vi "Workspace Tool with Event Messages - Starting point.vi"() -> ()   [LabVIEW 2016]
uses:
  NationalInstruments.VeriStand.SystemStorageUI
  NationalInstruments.VeriStand.SystemStorage
  <vilib>/NI Veristand/Templates/Workspace Tool Support/Workspace Tool Message Bus.ctl
  <vilib>/NI Veristand/Templates/Workspace Tool Support/Workspace Tool Message (String).ctl
  <vilib>/NI Veristand/Templates/Workspace Tool Support/Workspace Tool Response (String).ctl
  <vilib>/NI Veristand/Templates/Workspace Tool Support/Workspace Tool Message (Byte Array).ctl
  <vilib>/NI Veristand/Templates/Workspace Tool Support/Workspace Tool Response (Byte Array).ctl
  <vilib>/NI Veristand/Execution/Workspace/NI VeriStand - Get Multiple Channel Values.vi
  <vilib>/NI VeriStand/Execution/Workspace/NI_VS Workspace ExecutionAPI.lvlib
  <vilib>/NI Veristand/UI Controls/Single Node Browser/NI_VS UI Single Node Browser.lvlib
  <vilib>/NI VeriStand/Templates/Workspace Tool Support/NI VeriStand - Workspace Tool Support.lvlib
  <vilib>/NI Veristand/UI Controls/System Definition Tree/NI_VS UI System Tree.lvlib
panel:
  out "x+1":i32
  out "size(s)":i32
  out "types":i32[](array[ring]) items=["K_STRING", "K_BOOL", "K_I32", "K_U32", "K_DOUBLE", "K_U64", "K_VARIANT", "K_DEPENDENTFILE", "K_DEPENDENTNODE", "K_DATASOURCENODE", "K_U16", "K_DBLARR", "K_U32ARR", "K_I32ARR", "K_STRINGARR", "K_DICTIONARY", "K_DICTIONARYARR", "K_BINARYSTRING", "K_I16", "K_I64", "K_BOOLARR", "K_U64ARR", "K_U16ARR", "K_I64ARR", "K_I16ARR"]
  out "names":string[](array[string])
  in  "NIVS.Message Bus":T1
  out "Byte Array Data":u8[](array[numeric])
  out "String Data":string
  in  "Stop":bool
  in  "NIVS.System Definition Root":refnum<k24>
  in  "Tree Browser":refnum<k24>(container)
  in  "NIVS.Project File Path":path
  in  "Single Node Browser":refnum<k24>(container)
  in  "NIVS.Workspace Event":refnum<event-registration>
  out "System Times":dbl[](array[numeric]) format="%<%H:%M:%S%3u>t"
  out "Targets":string[](array[string])
  in  "NIVS.Gateway IP Address":string
  in  "NIVS.INI File Path":path
  # "Use this example as a template to create custom tools for the NI VeriStand Workspace. This example shows the use of the NI VeriStand API and UI controls to set and get data.\n\nRun this example by adding this VI as a Workspace Tool item. For Help adding Workspace Tool items, please reference the NI VeriStand Help."
  # "This code is used to register events from the\nNI VeriStand - Send Workspace Tool Message VI"
  # "With the assistance of the NI VeriStand Execution API, a tool has access to streaming data running on the target."
  # "This is the file path to the VeriStand system definition file. You can read or write to the file using the System Definition API."
  # "This is the root reference to the active System Definition file. You could use this to read the configuration or populate a tree with channels. You are free to close this reference, but it will be closed for you if you don't."
  # "The SystemStorageUI .NET assembly provides controls to display data configured in the System Definition file."
  # "This is the IP Address of the VeriStand Gateway to which the Workspace is connected. Use this to open all the .NET Manager references. Usually the Gateway is running on localhost, but it could be running on a neighbor's machine."
  # "This registered string User Event is used to help instruct your tool to shut down when the Workspace is closing."
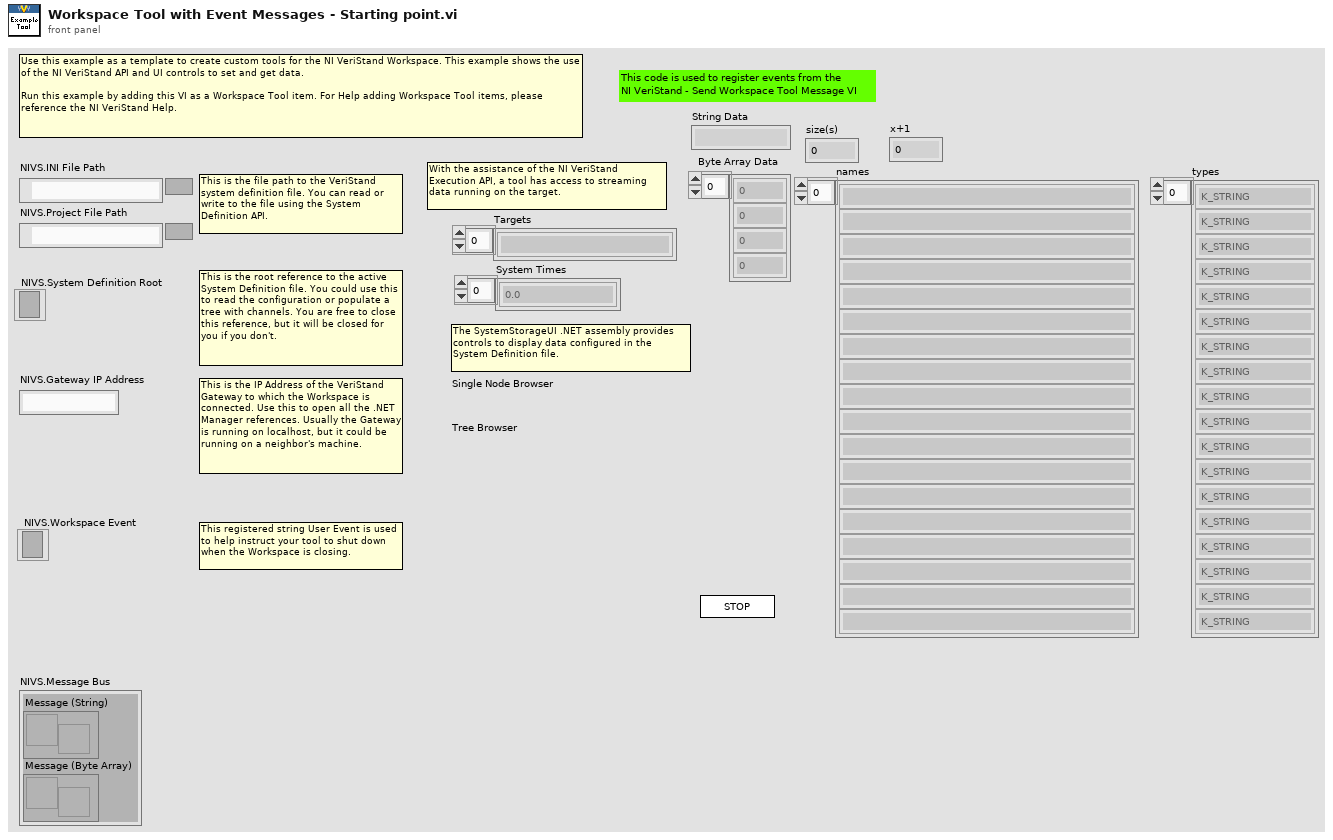
[diagram p1: front panel]
types:
  T1 = typedef "NI VeriStand - Workspace Tool Support.lvlib/Workspace Tool Message Bus.ctl" = cluster{"Message (String)":refnum<user-event>, "Message (Byte Array)":refnum<user-event>}
  T2 = typedef "NI_VS UI System Tree.lvlib/Callback Type.ctl" = cluster{"Net Callbacks":refnum<k27>[], "Event":T3}
  T3 = typedef "NI_VS UI System Tree.lvlib/Net Event Data Ref.ctl" = refnum<user-event>
  T4 = typedef "NI_VS UI Single Node Browser.lvlib/Callback Type.ctl" = cluster{"Net Callbacks":refnum<k27>[], "Event":refnum<user-event>}
  T5 = typedef "NI_VS Workspace ExecutionAPI.lvlib/WorkspaceAPI.ctl" = refnum<k24>
  T6 = typedef "NI_VS Workspace ExecutionAPI.lvlib/SystemStateEventRef.ctl" = cluster{"CustDatRef":refnum<user-event>, "EvtRef":refnum<k27>, "Target State User Event":refnum<user-event>}
  T7 = typedef "NI_VS Workspace ExecutionAPI.lvlib/SystemStateRegEventRef.ctl" = refnum<event-registration>
  T8 = cluster{"Event Registration Refnum":refnum<event-registration>, "NIVS.Workspace Event":refnum<event-registration>, "Event Registration Refnum":refnum<event-registration>, "Event Registration Refnum":refnum<event-registration>, "SystemChangeEventRef":T7}
  T9 = typedef "NI_VS UI Single Node Browser.lvlib/Node Ref.ctl" = refnum<k24>
  T10 = typedef "NI_VS UI System Tree.lvlib/Node Ref.ctl" = refnum<k24>
  T11 = typedef "NI VeriStand - Workspace Tool Support.lvlib/Workspace Tool Response (String).ctl" = cluster{"Response":string, "Error":errorcluster}
  T12 = typedef "NI VeriStand - Workspace Tool Support.lvlib/Workspace Tool Response (Byte Array).ctl" = cluster{"Response":u8[], "Error":errorcluster}
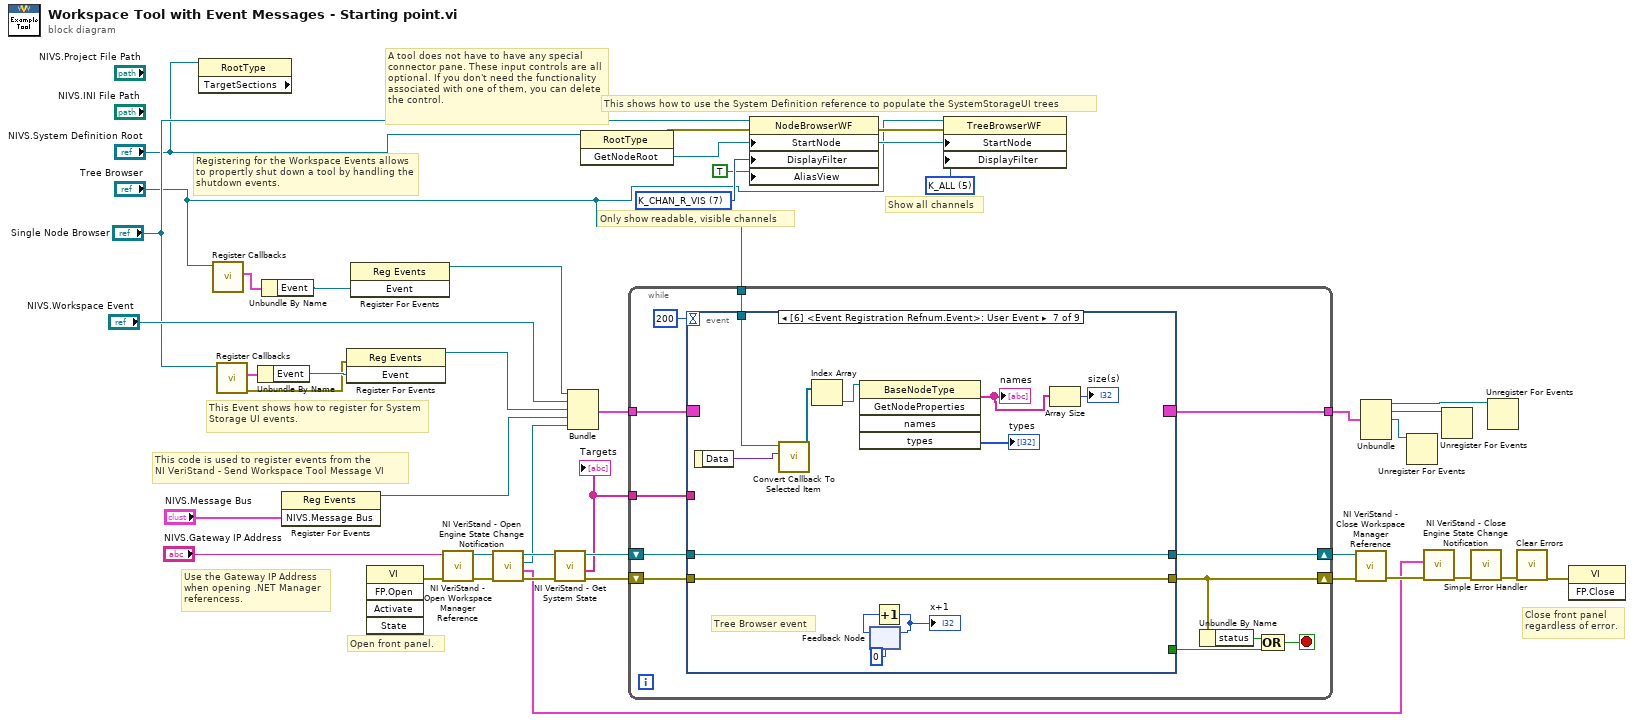
[diagram p0: block diagram]
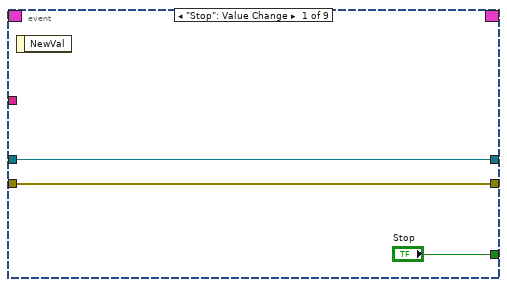
[diagram p2: hidden frame]
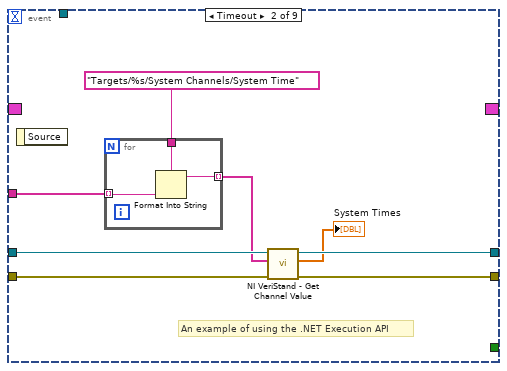
[diagram p3: hidden frame]
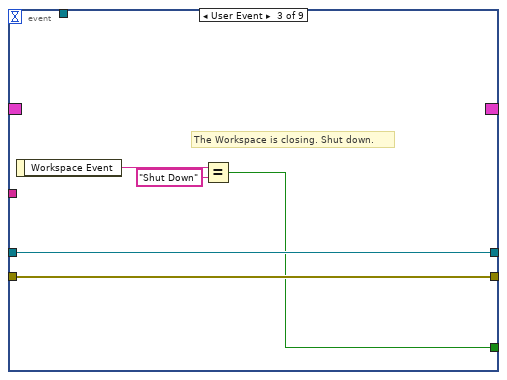
[diagram p4: hidden frame]
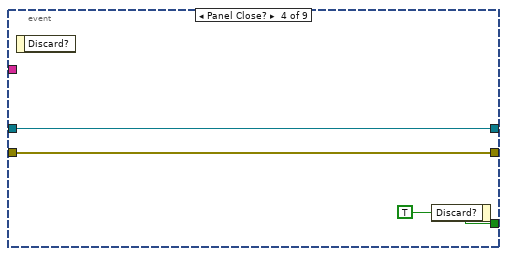
[diagram p5: hidden frame]
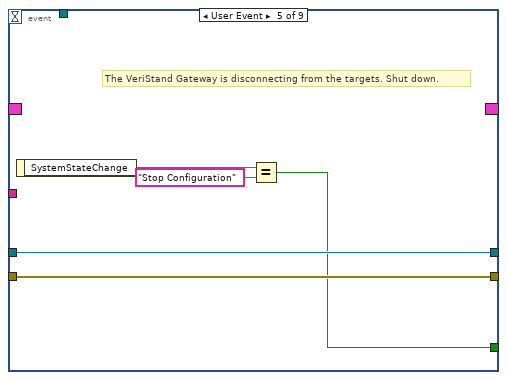
[diagram p6: hidden frame]
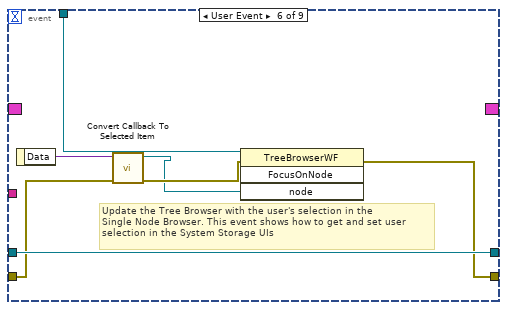
[diagram p7: hidden frame]
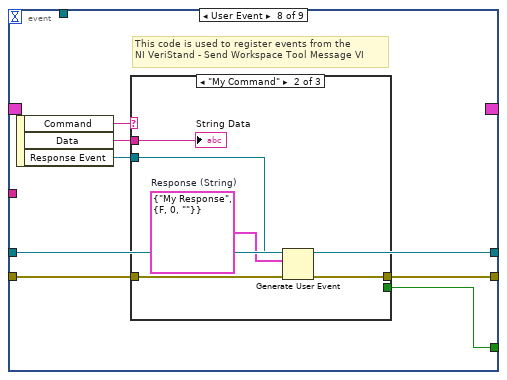
[diagram p8: hidden frame]
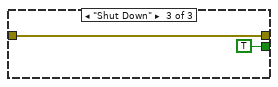
[diagram p10: hidden frame]
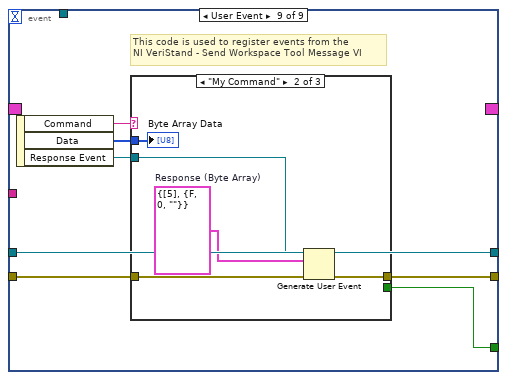
[diagram p11: hidden frame]
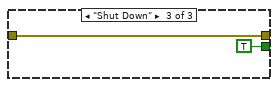
[diagram p13: hidden frame]
diagram:
  w15 = u8 7 items=["K_CHAN_R", "K_CHAN_W", "K_CHAN_RW", "K_CHAN_VOLT", "K_CHAN_FAULT", "K_ALL", "K_CUSTOM", "K_CHAN_R_VIS", "K_CHAN_W_VIS", "K_CHAN_RW_VIS", "K_CHAN_VOLT_VIS", "K_CHAN_FAULT_VIS"] ("DisplayFilter")
  w16 = u8 5 items=["K_CHAN_R", "K_CHAN_W", "K_CHAN_RW", "K_CHAN_VOLT", "K_CHAN_FAULT", "K_ALL", "K_CUSTOM", "K_CHAN_R_VIS", "K_CHAN_W_VIS", "K_CHAN_RW_VIS", "K_CHAN_VOLT_VIS", "K_CHAN_FAULT_VIS"] ("DisplayFilter")
  # "This code is used to register events from the\nNI VeriStand - Send Workspace Tool Message VI"
  # "Show all channels"
  # "Only show readable, visible channels"
  # "This Event shows how to register for System Storage UI events."
  # "Use the Gateway IP Address when opening .NET Manager referencess."
  # "A tool does not have to have any special connector pane. These input controls are all optional. If you don't need the functionality associated with one of them, you can delete the control."
  # "This shows how to use the System Definition reference to populate the SystemStorageUI trees"
  # "Registering for the Workspace Events allows to propertly shut down a tool by handling the shutdown events."
  # "Close front panel\nregardless of error."
  # "Open front panel."
  n1 = property class="RootType" props=["TargetSections"](reference="NIVS.System Definition Root") -> ()  [unwired: 1 in, 3 out]
  n2 = call <vilib>:"Register Callbacks.vi"("System Definition Tree"="Tree Browser") -> ("Callbacks"=w4:T2)  [unwired: 8 in, 2 out]
  n3 = call <vilib>:"Register Callbacks.vi"("Single Node Browser"="Single Node Browser") -> ("error out"=w10:errorcluster, "Callbacks"=w12:T4)  [unwired: 8 in, 1 out]
  n4 = Unbundle By Name(w12) -> ("Event"=w11:refnum<user-event>)
  n5 = Unbundle By Name(w4) -> ("Event"=w3:T3)
  n6 = register-events("NIVS.Message Bus") -> (reference out=w7:refnum<event-registration>)  [unwired: 2 in, 1 out]
  n7 = register-events(error in=w10, w11) -> (reference out=w17:refnum<event-registration>)  [unwired: 1 in, 1 out]
  n8 = register-events(w3) -> (reference out=w2:refnum<event-registration>)  [unwired: 2 in, 1 out]
  n9 = invoke class="VI" method="FP.Open"() -> (error out=w24:errorcluster)  [unwired: 5 in, 4 out]
  n10 = call <vilib>:"NI VeriStand - Open Workspace Manager Reference.vi"("error in (no error)"=w24, "Gateway IP Address (\"\": localhost)"="NIVS.Gateway IP Address") -> ("error out"=w35:errorcluster, "WorkspaceManager"=w36:T5)  [unwired: 8 in]
  n11 = call <vilib>:"NI VeriStand - Open Engine State Change Notification.vi"("error in (no error)"=w35, "WorkspaceManager in"=w36) -> ("error out"=w40:errorcluster, "SystemStateRefs"=w29:T6, "SystemChangeEventRef"=w8:T7, "WorkspaceManager out"=w41:T5)  [unwired: 6 in]
  n12 = call <vilib>:"NI VeriStand - Get System State.vi"("error in (no error)"=w40, "WorkspaceManager in"=w41) -> ("error out"=w27:errorcluster, "Targets"=w26:string[], "WorkspaceManager  out"=w28:T5)  [unwired: 5 in, 2 out]
  "Targets" <- w26
  n13 = Bundle("Event Registration Refnum"=w2, "NIVS.Workspace Event"="NIVS.Workspace Event", "Event Registration Refnum"=w17, "Event Registration Refnum"=w7, "SystemChangeEventRef"=w8) -> (w34:T8)  [unwired: 1 in]
  n14 = invoke class="RootType" method="GetNodeRoot"(reference="NIVS.System Definition Root") -> (error out=w18:errorcluster, "GetNodeRoot"=w19:refnum<k24>)  [unwired: 2 in, 1 out]
  n15 = while {
    tunnel: w34 -> [w53]
    tunnel: [w52] -> w33
    shift-right: [w45] -> w37
    shift-left: w27 -> [w50]
    shift-right: [w49] -> w38
    shift-left: w28 -> [w51]
    tunnel: w26 -> [w47]
    tunnel: "Tree Browser" -> [w42]
    stop <- w43 stop-if-true
    n16 = event shown="[6] <Event Registration Refnum.Event>: User Event" {
      selector: w53 -> [_ _ _ _ _ _ _ _ _]
      dyn-events: [_ _ _ _ _ _ _ _ _] -> w52
      timeout: 200 -> [_ _ _ _ _ _ _ _ _]
      tunnel: ["Stop" _ w68 w73 w76 _ _ w103 w118] -> w44
      tunnel: w51 -> [w55 w64 w71 w74 w79 w87 w98 w106 w121]
      tunnel: w50 -> [w56 w63 w72 w75 w80 w84 w99 w105 w120]
      tunnel: [w56 w58 w72 w75 w80 w82 w99 w102 w117] -> w45
      tunnel: [w55 w59 w71 w74 w79 w87 w98 w106 w121] -> w49
      tunnel: w47 -> [_ w62 _ _ _ _ _ _ _]
      tunnel: w42 -> [_ _ _ _ _ w86 w94 _ _]
      event "Stop": Value Change {
        n17 = event-data() -> ()  [unwired: 1 in, 1 out]
      }
      event Timeout {
        # "An example of using the .NET Execution API"
        n18 = event-data() -> ()  [unwired: 1 in, 1 out]
        n19 = for {
          tunnel: w62 -> [w66] mode=indexing
          tunnel: "Targets/%s/System Channels/System Time" ("format string") -> [w67]
          tunnel: [w65] -> w60 mode=indexing
          n20 = Format Into String(format string=w67, w66) -> (resulting string=w65:string)  [unwired: 2 in, 1 out]
        }
        n21 = call-poly <vilib>:"NI VeriStand - Get Channel Value.vi"("error in (no error)"=w63, "Channels"=w60, "WorkspaceManager in"=w64) -> ("error out"=w58:errorcluster, "Values"=→"System Times":dbl[], "WorkspaceManager out"=w59:T5)  [unwired: 6 in]
      }
      event User Event {
        # "The Workspace is closing. Shut down."
        n22 = event-data() -> ("Workspace Event"=w70:string)  [unwired: 1 in]
        n23 = Equal?(x=w70, y="Shut Down") -> (x = y?=w68:bool)
      }
      event Panel Close? {
        w73 = TRUE ("Discard?")
        n24 = event-data() -> ()  [unwired: 1 in, 1 out]
        n25 = event-data("Discard?"=w73) -> ()  [unwired: 1 in, 1 out]
      }
      event User Event {
        # "The VeriStand Gateway is disconnecting from the targets. Shut down."
        n26 = event-data() -> ("SystemStateChange"=w78:string)  [unwired: 1 in]
        n27 = Equal?(x=w78, y="Stop Configuration") -> (x = y?=w76:bool)
      }
      event User Event {
        # "Update the Tree Browser with the user's selection in the\nSingle Node Browser. This event shows how to get and set user\nselection in the System Storage UIs"
        n28 = event-data() -> ("Data"=w85:variant)  [unwired: 1 in]
        n29 = call <vilib>:"Convert Callback To Selected Item.vi"("error in"=w84, "Data"=w85) -> ("error out"=w83:errorcluster, "Selected Item"=w81:T9)  [unwired: 8 in]
        n30 = invoke class="TreeBrowserWF" method="FocusOnNode"(reference=w86, error in=w83, "node"=w81) -> (error out=w82:errorcluster)  [unwired: 1 in, 3 out]
      }
      event User Event {
        # "Tree Browser event"
        n31 = event-data() -> ("Data"=w95:variant)  [unwired: 1 in]
        n32 = call <vilib>:"Convert Callback To Selected Item.vi"("Data"=w95, "SystemDefinitionBrowser Ref"=w94) -> ("Selected Item"=w91:T10[])  [unwired: 8 in, 1 out]
        n33 = Index Array(array=w91) -> (element=w89:T10)  [unwired: 1 in]
        n34 = invoke class="BaseNodeType" method="GetNodeProperties"(reference=w89) -> ("names"=w90:string[], "types"=→"types":i32[])  [unwired: 4 in, 3 out]
        "names" <- w90
        n35 = feedback #1(0) -> (w88:i32)
        n36 = Increment(x=w88) -> (x+1=w97:i32)
        "x+1" <- w97
        n37 = feedback-in #1(w97) -> ()
        n38 = Array Size(array=w90) -> (size(s)=→"size(s)":i32)
      }
      event User Event {
        # "This code is used to register events from the\nNI VeriStand - Send Workspace Tool Message VI"
        n39 = event-data() -> ("Command"=w104:string, "Data"=w101:string, "Response Event"=w100:refnum<user-event>)  [unwired: 1 in]
        n40 = case shown="\"My Command\"" w104 {
          tunnel: w105 -> [w107 w111 w113]
          tunnel: [_ _ TRUE] -> w103
          tunnel: [w107 w110 w113] -> w102
          tunnel: w101 -> [_ w109 _]
          tunnel: w100 -> [_ w108 _]
          frame Default {
          }
          frame "My Command" {
            w112 = T11 {"Response"="My Response", "Error"={"status"=FALSE, "code"=0, "source"=""}}  # Response (String)
            n41 = Generate User Event(user event=w108, event data cluster=w112, error in=w111) -> (error out=w110:errorcluster)  [unwired: 1 in, 1 out]
            "String Data" <- w109
          }
          frame "Shut Down" {
          }
        }
      }
      event User Event {
        # "This code is used to register events from the\nNI VeriStand - Send Workspace Tool Message VI"
        n42 = event-data() -> ("Command"=w119:string, "Data"=w116:u8[], "Response Event"=w115:refnum<user-event>)  [unwired: 1 in]
        n43 = case shown="\"My Command\"" w119 {
          tunnel: w120 -> [w122 w127 w128]
          tunnel: [_ _ TRUE] -> w118
          tunnel: [w122 w126 w128] -> w117
          tunnel: w116 -> [_ w124 _]
          tunnel: w115 -> [_ w125 _]
          frame Default {
          }
          frame "My Command" {
            w123 = T12 {"Response"=[5], "Error"={"status"=FALSE, "code"=0, "source"=""}}  # Response (Byte Array)
            n44 = Generate User Event(user event=w125, event data cluster=w123, error in=w127) -> (error out=w126:errorcluster)  [unwired: 1 in, 1 out]
            "Byte Array Data" <- w124
          }
          frame "Shut Down" {
          }
        }
      }
    }
    n45 = Unbundle By Name(w45) -> ("status"=w46:bool)
    n46 = Compound Arithmetic op=OR(w46, w44) -> (w43:bool)
  }
  n47 = property class="NodeBrowserWF"(reference="Single Node Browser", error in=w18, "StartNode"=w19, "DisplayFilter"=w15, "AliasView"=TRUE) -> (error out=w20:errorcluster)  [unwired: 1 out]
  n48 = property class="TreeBrowserWF"(reference="Tree Browser", error in=w20, "StartNode"=w19, "DisplayFilter"=w16) -> ()  [unwired: 2 out]
  n49 = call <vilib>:"NI VeriStand - Close Workspace Manager Reference.vi"("error in (no error)"=w37, "WorkspaceManager"=w38) -> ("error out"=w30:errorcluster)  [unwired: 9 in]
  n50 = Unbundle(w33) -> ("Event Registration Refnum"=w31:refnum<event-registration>, "NIVS.Workspace Event"=w32:refnum<event-registration>, "Event Registration Refnum"=w1:refnum<event-registration>)  [unwired: 2 out]
  n51 = Unregister For Events(event registration refnum=w1) -> ()  [unwired: 1 in, 1 out]
  n52 = call <vilib>:"NI VeriStand - Close Engine State Change Notification.vi"("error in (no error)"=w30, "SystemStateRefs"=w29) -> ("error out"=w23:errorcluster)  [unwired: 9 in]
  n53 = Unregister For Events(event registration refnum=w32) -> ()  [unwired: 1 in, 1 out]
  n54 = call <vilib>:"Simple Error Handler.vi"("error in (no error)"=w23) -> ("error out"=w22:errorcluster)  [unwired: 4 in, 4 out]
  n55 = Unregister For Events(event registration refnum=w31) -> ()  [unwired: 1 in, 1 out]
  n56 = call <vilib>:"Clear Errors.vi"("error in (no error)"=w22) -> ("error out"=w21:errorcluster)  [unwired: 5 in, 1 out]
  n57 = invoke class="VI" method="FP.Close"(error in=w21) -> ()  [unwired: 2 in, 3 out]
